vi "Octave Display (line).vi"(1 "bandedge frequencies [Hz]":T1(array[cluster]) {"midband" format="%.2f"; "f high" format="%.2f"; "f low" format="%.2f"}, 2 "nominal frequencies [Hz]":dbl[](array[numeric]) format="%.2f", 3 "band power [dB EU]":dbl[](array[numeric]) format="%.2f") -> (0 "octave display":cluster{dbl[], dbl[]} {"?" format="%.2f"; "?" format="%.2f"})   [LabVIEW 2017]
doc: "Converts the result of any fractional-octave analysis into an octave spectrum to display as a line graph. Use this VI to display multiple octave spectra on the same graph."
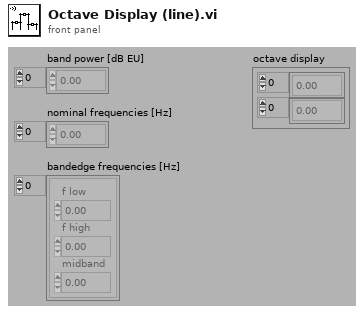
[diagram p1: front panel]
types:
  T1 = cluster{"f low":dbl, "f high":dbl, "midband":dbl}[]
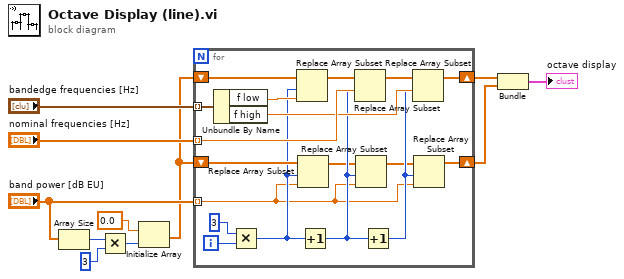
[diagram p0: block diagram]
diagram:
  n1 = Array Size(array="band power [dB EU]") -> (size(s)=w6:i32)
  n2 = Multiply(x=w6, y=3) -> (x*y=w4:i32)
  n3 = Initialize Array(0.0, w4) -> (w2:dbl[])
  n4 = for {
    tunnel: "bandedge frequencies [Hz]" -> [w29] mode=indexing
    tunnel: "nominal frequencies [Hz]" -> [w24] mode=indexing
    tunnel: "band power [dB EU]" -> [w12] mode=indexing
    shift-right: [w20] -> w9
    shift-left: w2 -> [w26]
    shift-right: [w13] -> w8
    shift-left: w2 -> [w19]
    i -> [w28]
    n5 = Unbundle By Name(w29) -> ("f low"=w25:dbl, "f high"=w23:dbl)
    n6 = Multiply(x=3, y=w28) -> (x*y=w18:i32)
    n7 = Replace Array Subset(array=w26, new element=w25, index=w18) -> (w22:dbl[])
    n8 = Replace Array Subset(array=w19, new element=w12, index=w18) -> (w15:dbl[])
    n9 = Increment(x=w18) -> (x+1=w17:i32)
    n10 = Replace Array Subset(array=w22, new element=w24, index=w17) -> (w21:dbl[])
    n11 = Replace Array Subset(array=w15, new element=w12, index=w17) -> (w14:dbl[])
    n12 = Increment(x=w17) -> (x+1=w16:i32)
    n13 = Replace Array Subset(array=w21, new element=w23, index=w16) -> (w20:dbl[])
    n14 = Replace Array Subset(array=w14, new element=w12, index=w16) -> (w13:dbl[])
  }
  n15 = Bundle(w9, w8) -> (→"octave display":cluster{dbl[], dbl[]})  [unwired: 1 in]
